vi "Get All Enpoint Configurations.vi"(8 "error in (no error)":errorcluster, 11 "Endpoint Config Section Ref in":T3 format="%.0x") -> (0 "error out":errorcluster, 1 "Endpoints found":bool, 2 "All Endpoint Configurations":T1[](array[typedef]), 3 "Endpoint Config Section Ref out":T3 format="%.0x")   [LabVIEW 2017, in "SLSC Switch Scripting.lvlib"]
uses:
  SLSC Switch Scripting.lvlib
  <vilib>/NI Veristand/Custom Device API/Custom Device Item Ref.ctl
  Endpoint Configuration Cluster.ctl
  Endpoint Configuration.ctl
  <vilib>/NI VeriStand/Custom Device API/Custom Device API.lvlib
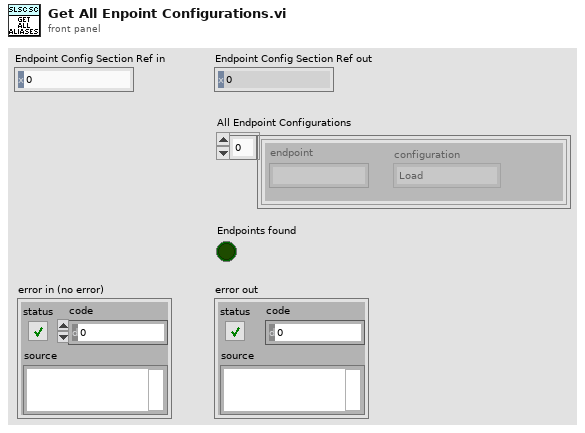
[diagram p1: front panel]
types:
  T1 = typedef "SLSC Switch Scripting.lvlib/Endpoint Configuration Cluster.ctl" = cluster{"endpoint":string, "configuration":T2}
  T2 = typedef "SLSC Switch Scripting.lvlib/Endpoint Configuration.ctl" = enum16{"Load", "Source", "Configuration"}
  T3 = typedef "Custom Device API.lvlib/Custom Device Item Ref.ctl" = u64
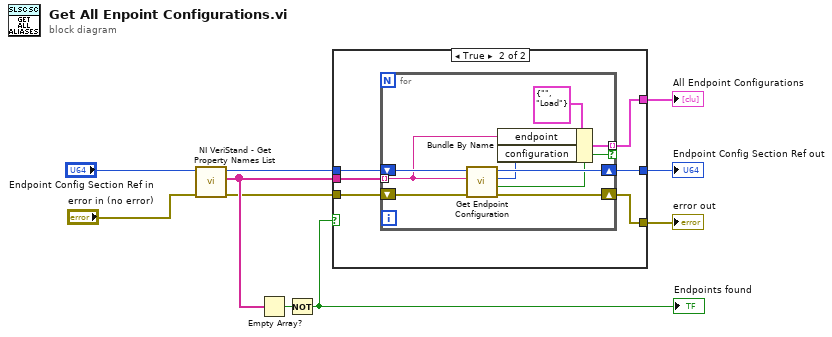
[diagram p0: block diagram]
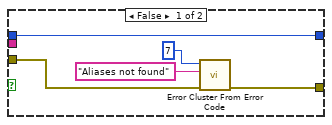
[diagram p2: hidden frame]
diagram:
  n1 = call <vilib>:"NI VeriStand - Get Property Names List.vi"("error in (no error)"="error in (no error)", "Item Ref in"="Endpoint Config Section Ref in") -> ("error out"=w8:errorcluster, "Property Names"=w9:string[], "Item Ref out"=w3:T3)  [unwired: 7 in]
  n2 = Empty Array?(array=w9) -> (empty?=w10:bool)
  n3 = Not(x=w10) -> (.not. x?=w1:bool)
  "Endpoints found" <- w1
  n4 = case shown="True" w1 {
    tunnel: w9 -> [_ w21]
    tunnel: w8 -> [w12 w20]
    tunnel: [_ w19] -> w6
    tunnel: [w11 w18] -> w5
    tunnel: w3 -> [w15 w17]
    tunnel: [w15 w16] -> w2
    frame False {
      n5 = call <vilib>:"Error Cluster From Error Code.vi"("error in (no error)"=w12, "error message (\"\")"="Aliases not found" ("error message (\"\")"), "error code (0)"=7) -> ("error out"=w11:errorcluster)  [unwired: 6 in]
    }
    frame True {
      n6 = for {
        tunnel: w21 -> [w26] mode=indexing
        shift-right: [w24] -> w18
        shift-left: w20 -> [w27]
        tunnel: [w30] -> w19 mode=indexing if=w23
        shift-right: [w28] -> w16
        shift-left: w17 -> [w29]
        n7 = call "Get Endpoint Configuration.vi"("error in (no error)"=w27, "Endpoint"=w26, "Endpoint Config Section Ref in"=w29) -> ("error out"=w24:errorcluster, "Endpoint found"=w23:bool, "Configuration Type"=w25:T2, "Endpoint Config Section Ref out"=w28:T3)  [unwired: 5 in]
        n8 = Bundle By Name(cluster=T1 {"endpoint"="", "configuration"=enum."Load"} ("Connection"), "endpoint"=w26, "configuration"=w25) -> (w30:T1)
      }
    }
  }
  "error out" <- w5
  "Endpoint Config Section Ref out" <- w2
  "All Endpoint Configurations" <- w6
